vi "trio_move.vi"(6 "Axis enable":bool[](array[boolean])=[TRUE, TRUE, TRUE, TRUE], 7 "Timeout (ms)":u32, 8 "error in":errorcluster, 9 "Axis positions":dbl[](array[numeric])=[0.0, 0.0, 0.0, 0.0], 10 "Absolute":bool=TRUE, 11 "Trio handle":refnum<k7>) -> (0 "error out":errorcluster, 1 "Motion error":dbl[](array[numeric]))   [LabVIEW 2024]
uses:
  <instrlib>/Trio Motion/Trio Motion Library.lvlib
panel:
  out "Final positions":dbl[](array[numeric])
  in  "Following threshold":dbl=16.0
  out "Reverse limit":bool[](array[boolean])
  out "Forward limit":bool[](array[boolean])
  # "How long to wait for motion to complete."
  # "The purposes of axis enable is to allow a subset of axes to be driven in absolute position mode without changing (or knowing) the positions of the other axes.   Being disabled just means that we don't want to move that axis, not that we want it powered down."
  # "Error if the motion deviates from command  by more than this many microsteps"
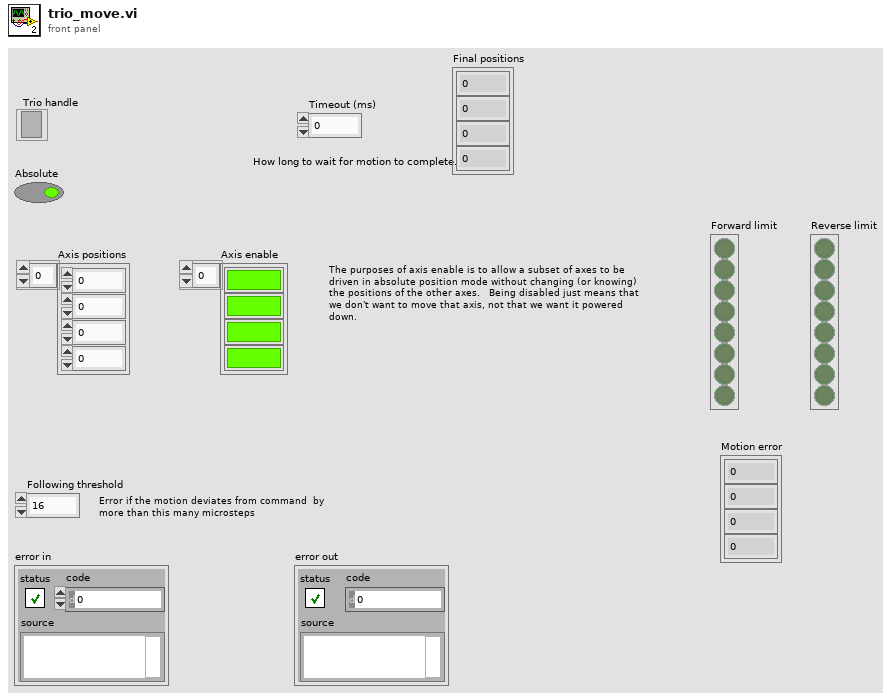
[diagram p1: front panel]
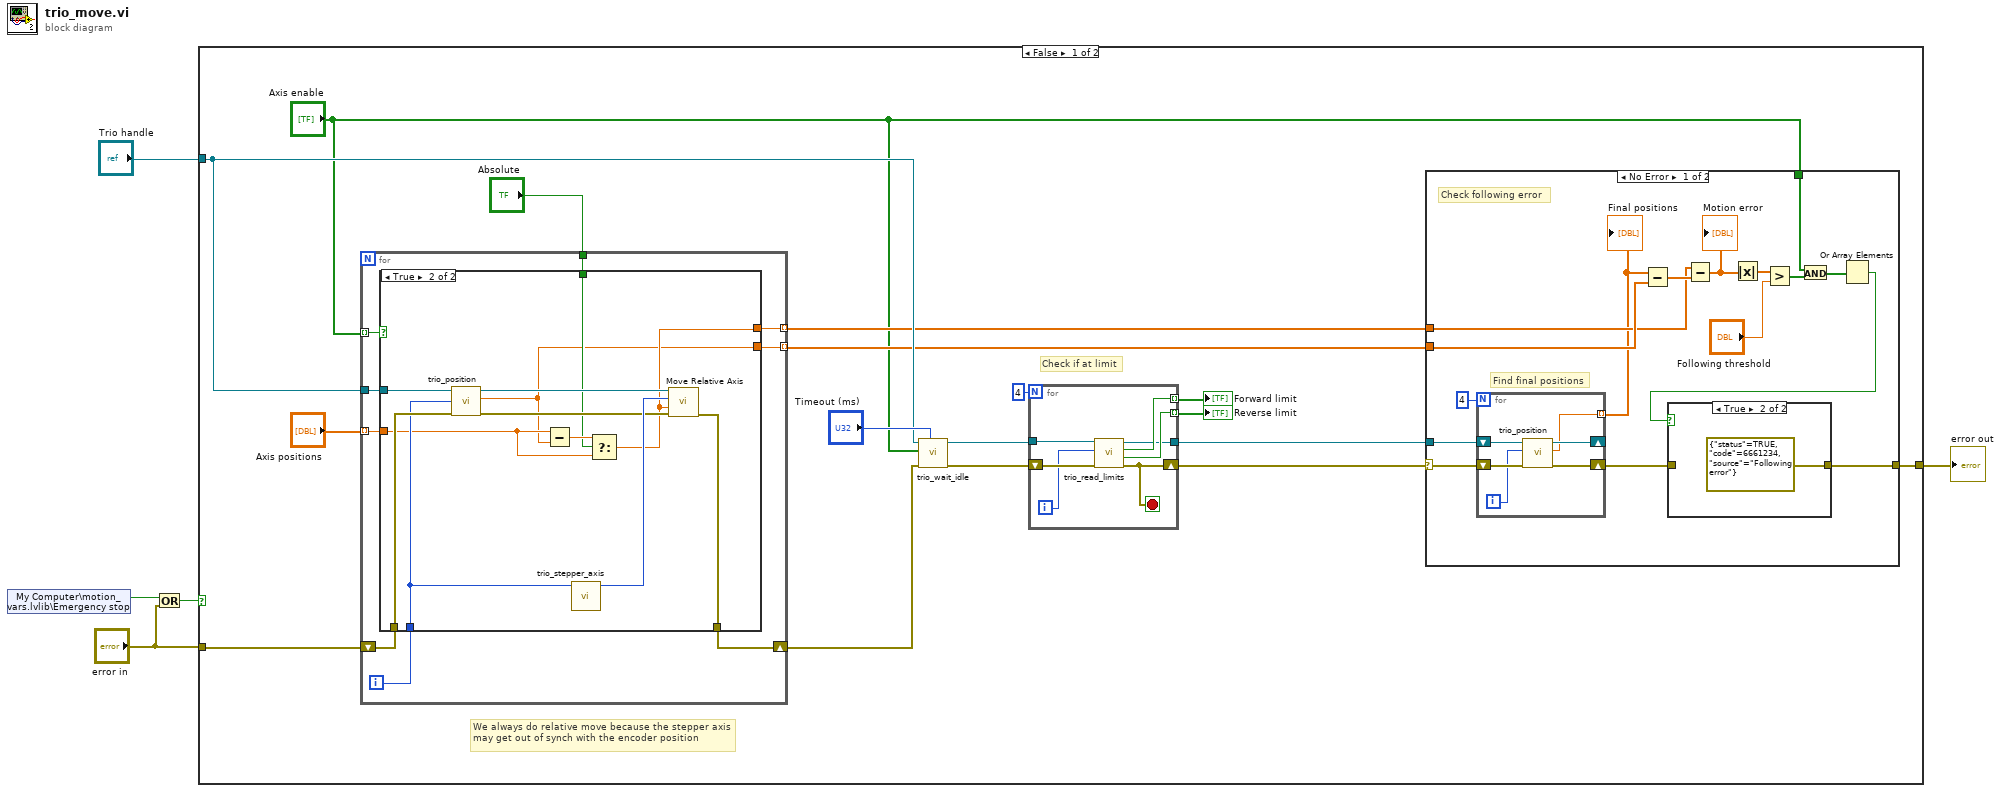
[diagram p0: block diagram]
diagram:
  n1 = shared-variable "My Computer\\motion_vars.lvlib\\Emergency stop"() -> (w4:bool)  [unwired: 1 in, 1 out]
  n2 = Or(x=w4, y="error in") -> (x .or. y?=w2:bool)
  n3 = case shown="False" w2 {
    tunnel: "error in" -> [w21 w77]
    tunnel: [w7 w77] -> w5
    tunnel: "Trio handle" -> [w14 _]
    frame False {
      # "Check if at limit"
      # "We always do relative move because the stepper axis may get out of synch with the encoder position"
      n4 = for {
        tunnel: "Axis enable" -> [w62] mode=indexing
        tunnel: "Axis positions" -> [w61] mode=indexing
        shift-right: [w60] -> w19
        shift-left: w21 -> [w63]
        tunnel: "Absolute" -> [w58]
        tunnel: w14 -> [w57]
        tunnel: [w56] -> w12 mode=indexing
        tunnel: [w55] -> w13 mode=indexing
        i -> [w59]
        n5 = case shown="True" w62 {
          tunnel: w63 -> [w64 w74]
          tunnel: w59 -> [_ w72]
          tunnel: w61 -> [_ w67]
          tunnel: [w64 w75] -> w60
          tunnel: w58 -> [_ w68]
          tunnel: w57 -> [_ w76]
          tunnel: [_ w66] -> w56
          tunnel: [_ w65] -> w55
          frame False {
          }
          frame True {
            n6 = call "trio_position.vi"("error in"=w74, "Axis"=w72, "Trio handle"=w76) -> ("error out"=w71:errorcluster, "Position"=w65:dbl, "Handle out"=w70:refnum<k7>)  [unwired: 6 in]
            n7 = Subtract(x=w67, y=w65) -> (x-y=w69:dbl)
            n8 = call "trio_stepper_axis.vi"("Encoder axis"=w72) -> ("Stepper axis"=w73:i32)  [unwired: 10 in]
            n9 = Select(t=w69, s=w68, f=w67) -> (s? t:f=w66:dbl)
            n10 = call <instrlib>:"Move Relative Axis.vi"("error in (no error)"=w71, "Distance"=w66, "Axis (0)"=w73, "reference in"=w70) -> ("error out"=w75:errorcluster)  [unwired: 5 in, 2 out]
          }
        }
      }
      n11 = call "trio_wait_idle.vi"("Timeout"="Timeout (ms)", "error in"=w19, "Axis enable"="Axis enable", "Trio ref in"=w14) -> ("error out"=w10:errorcluster, "Trio ref out"=w8:refnum<k7>)  [unwired: 5 in, 1 out]
      n12 = for {
        N: 4 -> [_]
        tunnel: w8 -> [w53]
        tunnel: [w50] -> w17 mode=indexing
        tunnel: [w49] -> w16 mode=indexing
        shift-right: [w51] -> w9
        shift-left: w10 -> [w54]
        tunnel: [w48] -> w6
        i -> [w52]
        stop <- w51 stop-if-true
        n13 = call "trio_read_limits.vi"("error in (no error)"=w54, "Axis"=w52, "Trio ref in"=w53) -> ("error out"=w51:errorcluster, "Reverse Limit"=w50:bool, "Forward Limit"=w49:bool, "Trio ref out"=w48:refnum<k7>)  [unwired: 5 in]
      }
      "Forward limit" <- w16
      "Reverse limit" <- w17
      n14 = case shown="No Error" w9 {
        selector: w9 -> [w28 w47]
        tunnel: w13 -> [w37 _]
        tunnel: w12 -> [w35 _]
        tunnel: "Axis enable" -> [w30 _]
        tunnel: [w25 w47] -> w7
        tunnel: w6 -> [w24 _]
        frame No Error {
          # "Check following error"
          # "Find final positions"
          n15 = for {
            N: 4 -> [_]
            shift-right: [w45] -> _
            shift-left: w24 -> [w46]
            tunnel: [w42] -> w23 mode=indexing
            shift-right: [w41] -> w27
            shift-left: w28 -> [w44]
            i -> [w43]
            n16 = call "trio_position.vi"("error in"=w44, "Axis"=w43, "Trio handle"=w46) -> ("error out"=w41:errorcluster, "Position"=w42:dbl, "Handle out"=w45:refnum<k7>)  [unwired: 6 in]
          }
          "Final positions" <- w23
          n17 = Subtract(x=w23, y=w37) -> (x-y=w36:dbl[])
          n18 = Subtract(x=w35, y=w36) -> (x-y=w32:dbl[])
          "Motion error" <- w32
          n19 = Absolute Value(x=w32) -> (abs(x)=w33:dbl[])
          n20 = Greater?(x=w33, y="Following threshold") -> (0:w31:bool[])
          n21 = And(x=w30, y=w31) -> (x .and. y?=w29:bool[])
          n22 = Or Array Elements(Boolean array=w29) -> (logical OR=w26:bool)
          n23 = case shown="True" w26 {
            tunnel: [w39 errorcluster {"status"=TRUE, "code"=6661234, "source"="Following error"} ("error out")] -> w25
            tunnel: w27 -> [w39 _]
            frame False {
            }
            frame True {
            }
          }
        }
        frame Error {
        }
      }
    }
    frame True {
    }
  }
  "error out" <- w5
